vi "HumanDriveButtonBoxReef.vi"(6 "KL":bool, 7 "AB":bool, 8 "IJ":bool, 9 "GH":bool, 10 "EF":bool, 11 "CD":bool) -> (3 "DriveTraj?":bool)   [LabVIEW 2023]
uses:
  HumanBoxReefENUM.ctl
  HumanGlobal.vi
  <vilib>/Rock Robotics/WPI/ThirdParty/JAS_Junk/TrajLib/Trajectory_Library.lvlib
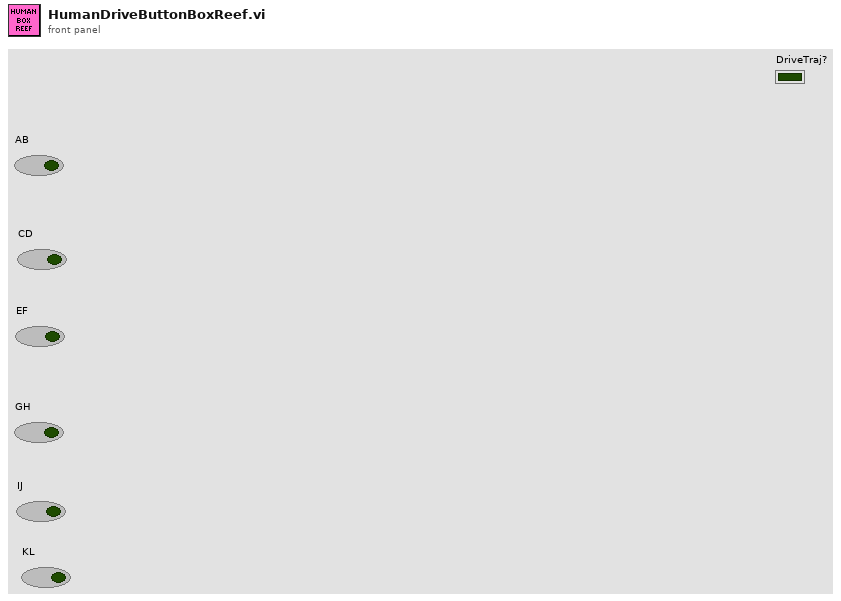
[diagram p1: front panel]
types:
  T1 = typedef "HumanBoxReefENUM.ctl" = enum16{"NoTraj", "A", "B", "C", "D", "E", "F", "G", "H", "I", "J", "K", "L"}
  T2 = typedef "WPI_DriverStationAllianceInfo.ctl" = enum16{"Red", "Blue", "Invalid"}
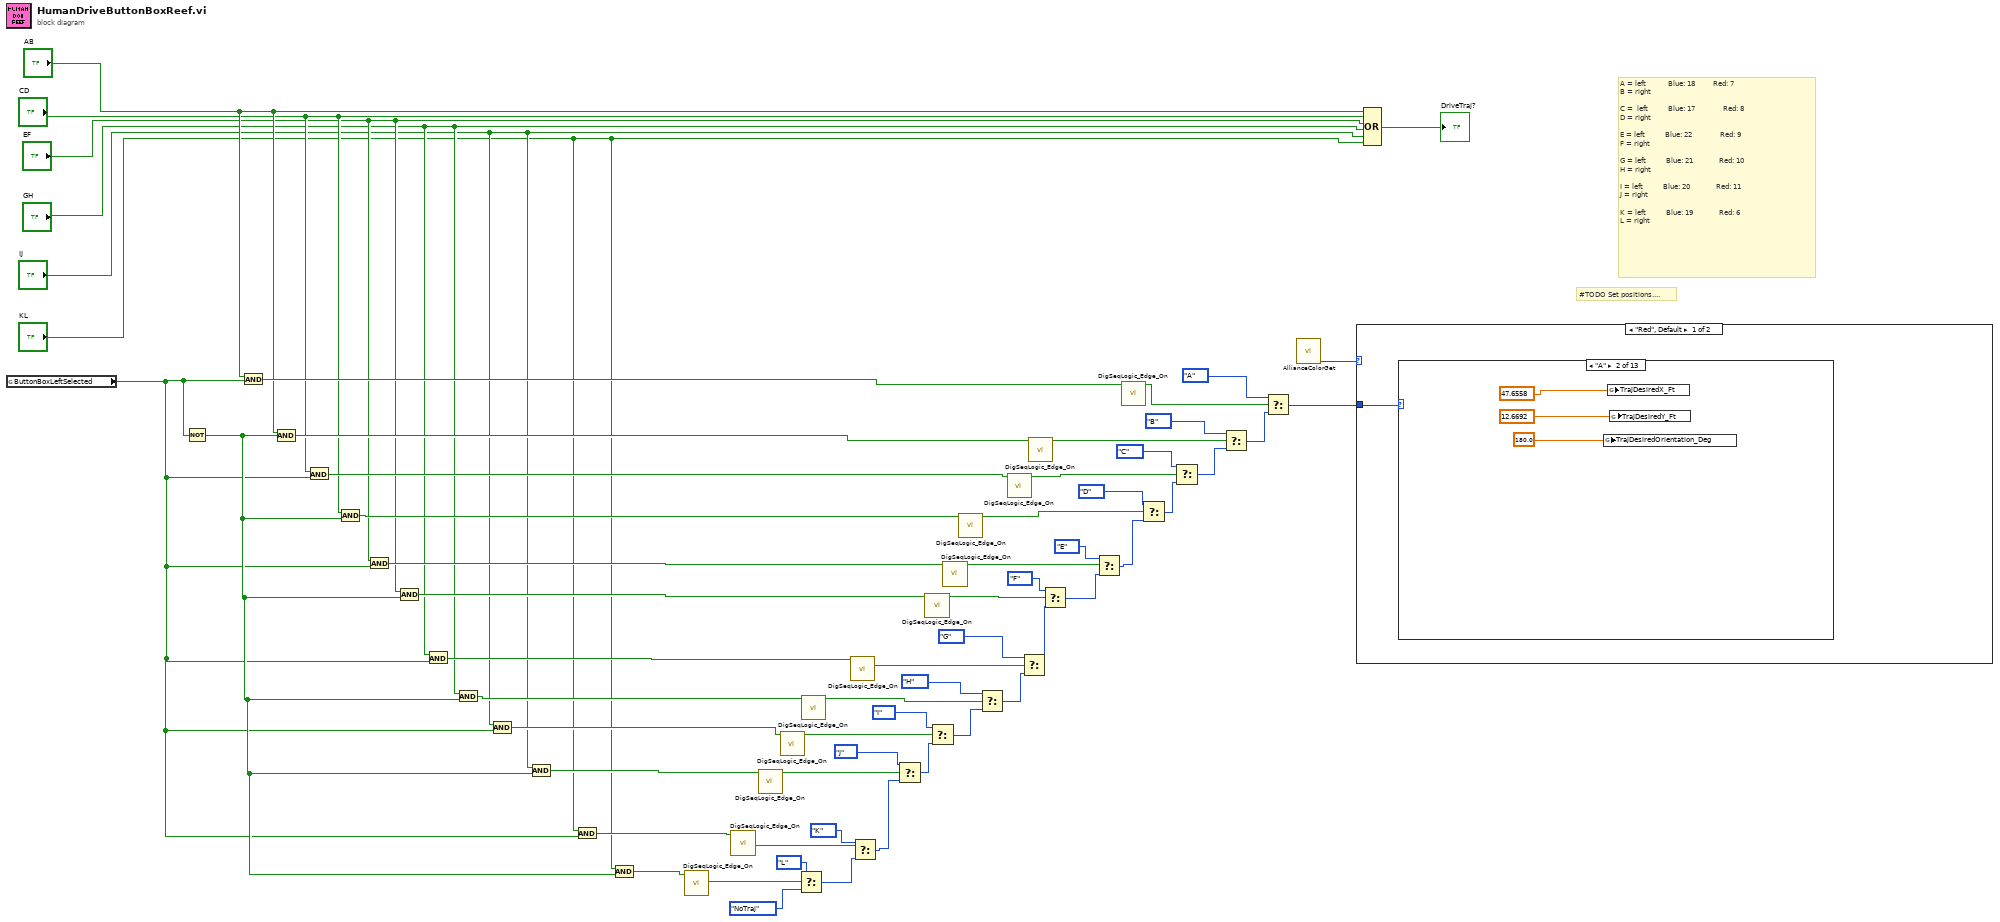
[diagram p0: block diagram]
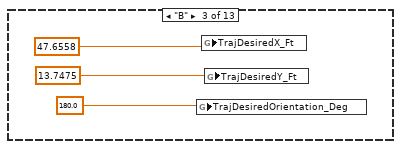
[diagram p3: hidden frame]
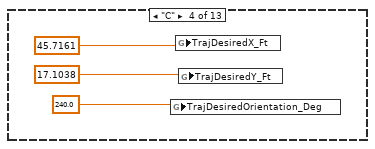
[diagram p4: hidden frame]
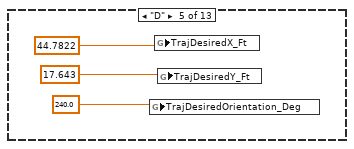
[diagram p5: hidden frame]
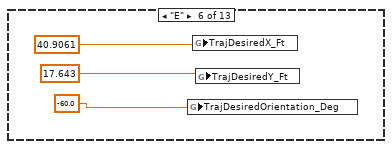
[diagram p6: hidden frame]
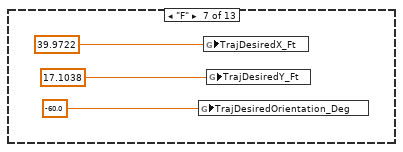
[diagram p7: hidden frame]
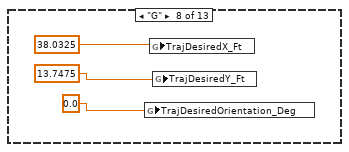
[diagram p8: hidden frame]
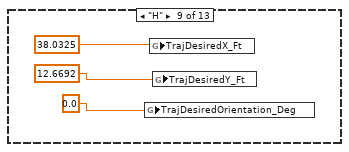
[diagram p9: hidden frame]
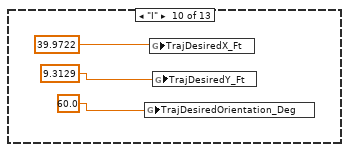
[diagram p10: hidden frame]
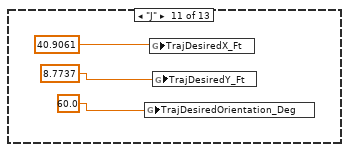
[diagram p11: hidden frame]
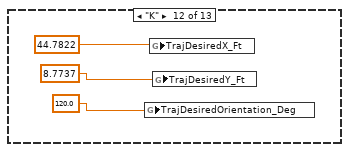
[diagram p12: hidden frame]
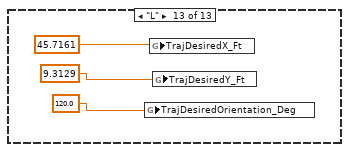
[diagram p13: hidden frame]
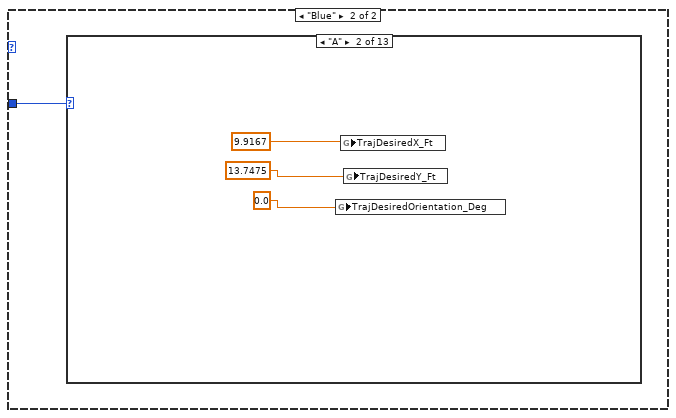
[diagram p14: hidden frame]
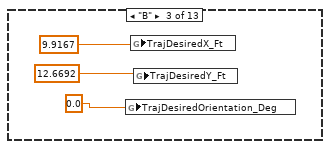
[diagram p16: hidden frame]
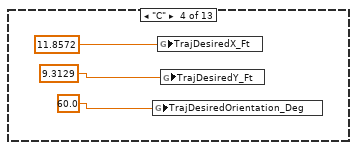
[diagram p17: hidden frame]
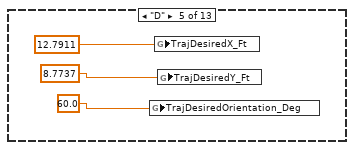
[diagram p18: hidden frame]
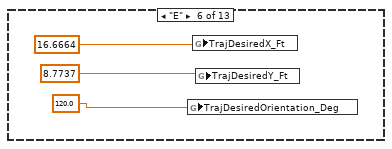
[diagram p19: hidden frame]
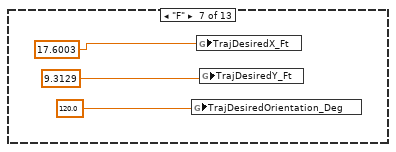
[diagram p20: hidden frame]
diagram:
  # "A = left           Blue: 18         Red: 7\nB = right\n\nC =  left          Blue: 17              Red: 8\nD = right\n\nE = left          Blue: 22              Red: 9\nF = right\n\nG = left          Blue: 21             Red: 10\nH = right\n\nI = left          Blue: 20             Red: 11\nJ = right\n\nK = left          Blue: 19             Red: 6\nL = right"
  # "#TODO Set positions...."
  n1 = global read "HumanGlobal.vi" "ButtonBoxLeftSelected"() -> (w1:bool)
  n2 = Not(x=w1) -> (.not. x?=w2:bool)
  n3 = And(x="AB", y=w1) -> (x .and. y?=w21:bool)
  n4 = And(x="AB", y=w2) -> (x .and. y?=w20:bool)
  n5 = And(x="CD", y=w1) -> (x .and. y?=w19:bool)
  n6 = And(x="CD", y=w2) -> (x .and. y?=w18:bool)
  n7 = And(x="EF", y=w1) -> (x .and. y?=w17:bool)
  n8 = And(x="EF", y=w2) -> (x .and. y?=w16:bool)
  n9 = And(x="GH", y=w1) -> (x .and. y?=w15:bool)
  n10 = And(x="GH", y=w2) -> (x .and. y?=w14:bool)
  n11 = And(x="IJ", y=w1) -> (x .and. y?=w13:bool)
  n12 = And(x="IJ", y=w2) -> (x .and. y?=w12:bool)
  n13 = And(x="KL", y=w1) -> (x .and. y?=w11:bool)
  n14 = And(x="KL", y=w2) -> (x .and. y?=w10:bool)
  n15 = call <vilib>:"DigSeqLogic_Edge_On.vi"("Input"=w10) -> ("On Edge"=w41:bool)  [unwired: 10 in]
  n16 = call <vilib>:"DigSeqLogic_Edge_On.vi"("Input"=w11) -> ("On Edge"=w35:bool)  [unwired: 10 in]
  n17 = call <vilib>:"DigSeqLogic_Edge_On.vi"("Input"=w12) -> ("On Edge"=w34:bool)  [unwired: 10 in]
  n18 = call <vilib>:"DigSeqLogic_Edge_On.vi"("Input"=w13) -> ("On Edge"=w33:bool)  [unwired: 10 in]
  n19 = Select(t=HumanBoxReefENUM."L", s=w41, f=HumanBoxReefENUM."NoTraj" ("t")) -> (s? t:f=w40:T1)
  n20 = call <vilib>:"DigSeqLogic_Edge_On.vi"("Input"=w14) -> ("On Edge"=w32:bool)  [unwired: 10 in]
  n21 = call <vilib>:"DigSeqLogic_Edge_On.vi"("Input"=w15) -> ("On Edge"=w31:bool)  [unwired: 10 in]
  n22 = Select(t=HumanBoxReefENUM."K", s=w35, f=w40) -> (s? t:f=w39:T1)
  n23 = Select(t=HumanBoxReefENUM."J", s=w34, f=w39) -> (s? t:f=w38:T1)
  n24 = call <vilib>:"DigSeqLogic_Edge_On.vi"("Input"=w16) -> ("On Edge"=w59:bool)  [unwired: 10 in]
  n25 = Select(t=HumanBoxReefENUM."I", s=w33, f=w38) -> (s? t:f=w37:T1)
  n26 = call <vilib>:"DigSeqLogic_Edge_On.vi"("Input"=w17) -> ("On Edge"=w53:bool)  [unwired: 10 in]
  n27 = call <vilib>:"DigSeqLogic_Edge_On.vi"("Input"=w18) -> ("On Edge"=w52:bool)  [unwired: 10 in]
  n28 = Select(t=HumanBoxReefENUM."H", s=w32, f=w37) -> (s? t:f=w36:T1)
  n29 = call <vilib>:"DigSeqLogic_Edge_On.vi"("Input"=w19) -> ("On Edge"=w51:bool)  [unwired: 10 in]
  n30 = Select(t=HumanBoxReefENUM."G", s=w31, f=w36) -> (s? t:f=w24:T1)
  n31 = call <vilib>:"DigSeqLogic_Edge_On.vi"("Input"=w20) -> ("On Edge"=w50:bool)  [unwired: 10 in]
  n32 = Select(t=HumanBoxReefENUM."F", s=w59, f=w24) -> (s? t:f=w58:T1)
  n33 = Select(t=HumanBoxReefENUM."E", s=w53, f=w58) -> (s? t:f=w57:T1)
  n34 = call <vilib>:"DigSeqLogic_Edge_On.vi"("Input"=w21) -> ("On Edge"=w22:bool)  [unwired: 10 in]
  n35 = Select(t=HumanBoxReefENUM."D", s=w52, f=w57) -> (s? t:f=w56:T1)
  n36 = Select(t=HumanBoxReefENUM."C", s=w51, f=w56) -> (s? t:f=w55:T1)
  n37 = Select(t=HumanBoxReefENUM."B", s=w50, f=w55) -> (s? t:f=w54:T1)
  n38 = Select(t=HumanBoxReefENUM."A", s=w22, f=w54) -> (s? t:f=w43:T1)
  n39 = call "AllianceColorGet.vi"() -> ("AllianceColor"=w42:T2)  [unwired: 11 in]
  n40 = case shown="\"Red\", Default" w42 {
    tunnel: w43 -> [w60 w97]
    frame "Red", Default {
      n41 = case shown="\"A\"" w60 {
        frame "NoTraj" {
        }
        frame "A" {
          n42 = global write "HumanGlobal.vi" "TrajDesiredOrientation_Deg"(180.0 ("TrajDesiredOrientation_Deg")) -> ()
          n43 = global write "HumanGlobal.vi" "TrajDesiredX_Ft"(47.6558 ("TrajDesiredX_Ft")) -> ()
          n44 = global write "HumanGlobal.vi" "TrajDesiredY_Ft"(12.6692 ("TrajDesiredY_Ft")) -> ()
        }
        frame "B" {
          n45 = global write "HumanGlobal.vi" "TrajDesiredOrientation_Deg"(180.0 ("TrajDesiredOrientation_Deg")) -> ()
          n46 = global write "HumanGlobal.vi" "TrajDesiredX_Ft"(47.6558 ("TrajDesiredX_Ft")) -> ()
          n47 = global write "HumanGlobal.vi" "TrajDesiredY_Ft"(13.7475 ("TrajDesiredY_Ft")) -> ()
        }
        frame "C" {
          n48 = global write "HumanGlobal.vi" "TrajDesiredOrientation_Deg"(240.0 ("TrajDesiredOrientation_Deg")) -> ()
          n49 = global write "HumanGlobal.vi" "TrajDesiredX_Ft"(45.7161 ("TrajDesiredX_Ft")) -> ()
          n50 = global write "HumanGlobal.vi" "TrajDesiredY_Ft"(17.1038 ("TrajDesiredY_Ft")) -> ()
        }
        frame "D" {
          n51 = global write "HumanGlobal.vi" "TrajDesiredOrientation_Deg"(240.0 ("TrajDesiredOrientation_Deg")) -> ()
          n52 = global write "HumanGlobal.vi" "TrajDesiredX_Ft"(44.7822 ("TrajDesiredX_Ft")) -> ()
          n53 = global write "HumanGlobal.vi" "TrajDesiredY_Ft"(17.643 ("TrajDesiredY_Ft")) -> ()
        }
        frame "E" {
          n54 = global write "HumanGlobal.vi" "TrajDesiredOrientation_Deg"(-60.0 ("TrajDesiredOrientation_Deg")) -> ()
          n55 = global write "HumanGlobal.vi" "TrajDesiredX_Ft"(40.9061 ("TrajDesiredX_Ft")) -> ()
          n56 = global write "HumanGlobal.vi" "TrajDesiredY_Ft"(17.643 ("TrajDesiredY_Ft")) -> ()
        }
        frame "F" {
          n57 = global write "HumanGlobal.vi" "TrajDesiredOrientation_Deg"(-60.0 ("TrajDesiredOrientation_Deg")) -> ()
          n58 = global write "HumanGlobal.vi" "TrajDesiredX_Ft"(39.9722 ("TrajDesiredX_Ft")) -> ()
          n59 = global write "HumanGlobal.vi" "TrajDesiredY_Ft"(17.1038 ("TrajDesiredY_Ft")) -> ()
        }
        frame "G" {
          n60 = global write "HumanGlobal.vi" "TrajDesiredOrientation_Deg"(0.0 ("TrajDesiredOrientation_Deg")) -> ()
          n61 = global write "HumanGlobal.vi" "TrajDesiredX_Ft"(38.0325 ("TrajDesiredX_Ft")) -> ()
          n62 = global write "HumanGlobal.vi" "TrajDesiredY_Ft"(13.7475 ("TrajDesiredY_Ft")) -> ()
        }
        frame "H" {
          n63 = global write "HumanGlobal.vi" "TrajDesiredOrientation_Deg"(0.0 ("TrajDesiredOrientation_Deg")) -> ()
          n64 = global write "HumanGlobal.vi" "TrajDesiredX_Ft"(38.0325 ("TrajDesiredX_Ft")) -> ()
          n65 = global write "HumanGlobal.vi" "TrajDesiredY_Ft"(12.6692 ("TrajDesiredY_Ft")) -> ()
        }
        frame "I" {
          n66 = global write "HumanGlobal.vi" "TrajDesiredOrientation_Deg"(60.0 ("TrajDesiredOrientation_Deg")) -> ()
          n67 = global write "HumanGlobal.vi" "TrajDesiredX_Ft"(39.9722 ("TrajDesiredX_Ft")) -> ()
          n68 = global write "HumanGlobal.vi" "TrajDesiredY_Ft"(9.3129 ("TrajDesiredY_Ft")) -> ()
        }
        frame "J" {
          n69 = global write "HumanGlobal.vi" "TrajDesiredOrientation_Deg"(60.0 ("TrajDesiredOrientation_Deg")) -> ()
          n70 = global write "HumanGlobal.vi" "TrajDesiredX_Ft"(40.9061 ("TrajDesiredX_Ft")) -> ()
          n71 = global write "HumanGlobal.vi" "TrajDesiredY_Ft"(8.7737 ("TrajDesiredY_Ft")) -> ()
        }
        frame "K" {
          n72 = global write "HumanGlobal.vi" "TrajDesiredOrientation_Deg"(120.0 ("TrajDesiredOrientation_Deg")) -> ()
          n73 = global write "HumanGlobal.vi" "TrajDesiredX_Ft"(44.7822 ("TrajDesiredX_Ft")) -> ()
          n74 = global write "HumanGlobal.vi" "TrajDesiredY_Ft"(8.7737 ("TrajDesiredY_Ft")) -> ()
        }
        frame "L" {
          n75 = global write "HumanGlobal.vi" "TrajDesiredOrientation_Deg"(120.0 ("TrajDesiredOrientation_Deg")) -> ()
          n76 = global write "HumanGlobal.vi" "TrajDesiredX_Ft"(45.7161 ("TrajDesiredX_Ft")) -> ()
          n77 = global write "HumanGlobal.vi" "TrajDesiredY_Ft"(9.3129 ("TrajDesiredY_Ft")) -> ()
        }
      }
    }
    frame "Blue" {
      n78 = case shown="\"A\"" w97 {
        frame "NoTraj" {
        }
        frame "A" {
          n79 = global write "HumanGlobal.vi" "TrajDesiredOrientation_Deg"(0.0 ("TrajDesiredOrientation_Deg")) -> ()
          n80 = global write "HumanGlobal.vi" "TrajDesiredX_Ft"(9.9167 ("TrajDesiredX_Ft")) -> ()
          n81 = global write "HumanGlobal.vi" "TrajDesiredY_Ft"(13.7475 ("TrajDesiredY_Ft")) -> ()
        }
        frame "B" {
          n82 = global write "HumanGlobal.vi" "TrajDesiredOrientation_Deg"(0.0 ("TrajDesiredOrientation_Deg")) -> ()
          n83 = global write "HumanGlobal.vi" "TrajDesiredX_Ft"(9.9167 ("TrajDesiredX_Ft")) -> ()
          n84 = global write "HumanGlobal.vi" "TrajDesiredY_Ft"(12.6692 ("TrajDesiredY_Ft")) -> ()
        }
        frame "C" {
          n85 = global write "HumanGlobal.vi" "TrajDesiredOrientation_Deg"(60.0 ("TrajDesiredOrientation_Deg")) -> ()
          n86 = global write "HumanGlobal.vi" "TrajDesiredX_Ft"(11.8572 ("TrajDesiredX_Ft")) -> ()
          n87 = global write "HumanGlobal.vi" "TrajDesiredY_Ft"(9.3129 ("TrajDesiredY_Ft")) -> ()
        }
        frame "D" {
          n88 = global write "HumanGlobal.vi" "TrajDesiredOrientation_Deg"(60.0 ("TrajDesiredOrientation_Deg")) -> ()
          n89 = global write "HumanGlobal.vi" "TrajDesiredX_Ft"(12.7911 ("TrajDesiredX_Ft")) -> ()
          n90 = global write "HumanGlobal.vi" "TrajDesiredY_Ft"(8.7737 ("TrajDesiredY_Ft")) -> ()
        }
        frame "E" {
          n91 = global write "HumanGlobal.vi" "TrajDesiredOrientation_Deg"(120.0 ("TrajDesiredOrientation_Deg")) -> ()
          n92 = global write "HumanGlobal.vi" "TrajDesiredX_Ft"(16.6664 ("TrajDesiredX_Ft")) -> ()
          n93 = global write "HumanGlobal.vi" "TrajDesiredY_Ft"(8.7737 ("TrajDesiredY_Ft")) -> ()
        }
        frame "F" {
          n94 = global write "HumanGlobal.vi" "TrajDesiredOrientation_Deg"(120.0 ("TrajDesiredOrientation_Deg")) -> ()
          n95 = global write "HumanGlobal.vi" "TrajDesiredX_Ft"(17.6003 ("TrajDesiredX_Ft")) -> ()
          n96 = global write "HumanGlobal.vi" "TrajDesiredY_Ft"(9.3129 ("TrajDesiredY_Ft")) -> ()
        }
        frame "G" {
          n97 = global write "HumanGlobal.vi" "TrajDesiredOrientation_Deg"(180.0 ("TrajDesiredOrientation_Deg")) -> ()
          n98 = global write "HumanGlobal.vi" "TrajDesiredX_Ft"(19.5408 ("TrajDesiredX_Ft")) -> ()
          n99 = global write "HumanGlobal.vi" "TrajDesiredY_Ft"(12.6692 ("TrajDesiredY_Ft")) -> ()
        }
        frame "H" {
          n100 = global write "HumanGlobal.vi" "TrajDesiredOrientation_Deg"(180.0 ("TrajDesiredOrientation_Deg")) -> ()
          n101 = global write "HumanGlobal.vi" "TrajDesiredX_Ft"(19.5408 ("TrajDesiredX_Ft")) -> ()
          n102 = global write "HumanGlobal.vi" "TrajDesiredY_Ft"(13.7475 ("TrajDesiredY_Ft")) -> ()
        }
        frame "I" {
          n103 = global write "HumanGlobal.vi" "TrajDesiredOrientation_Deg"(240.0 ("TrajDesiredOrientation_Deg")) -> ()
          n104 = global write "HumanGlobal.vi" "TrajDesiredX_Ft"(17.6003 ("TrajDesiredX_Ft")) -> ()
          n105 = global write "HumanGlobal.vi" "TrajDesiredY_Ft"(17.1038 ("TrajDesiredY_Ft")) -> ()
        }
        frame "J" {
          n106 = global write "HumanGlobal.vi" "TrajDesiredOrientation_Deg"(240.0 ("TrajDesiredOrientation_Deg")) -> ()
          n107 = global write "HumanGlobal.vi" "TrajDesiredX_Ft"(16.6664 ("TrajDesiredX_Ft")) -> ()
          n108 = global write "HumanGlobal.vi" "TrajDesiredY_Ft"(17.643 ("TrajDesiredY_Ft")) -> ()
        }
        frame "K" {
          n109 = global write "HumanGlobal.vi" "TrajDesiredOrientation_Deg"(-45.0 ("TrajDesiredOrientation_Deg")) -> ()
          n110 = global write "HumanGlobal.vi" "TrajDesiredX_Ft"(12.2739 ("TrajDesiredX_Ft")) -> ()
          n111 = global write "HumanGlobal.vi" "TrajDesiredY_Ft"(17.4236 ("TrajDesiredY_Ft")) -> ()
        }
        frame "L" {
          n112 = global write "HumanGlobal.vi" "TrajDesiredOrientation_Deg"(-45.0 ("TrajDesiredOrientation_Deg")) -> ()
          n113 = global write "HumanGlobal.vi" "TrajDesiredX_Ft"(11.5114 ("TrajDesiredX_Ft")) -> ()
          n114 = global write "HumanGlobal.vi" "TrajDesiredY_Ft"(16.6611 ("TrajDesiredY_Ft")) -> ()
        }
      }
    }
  }
  n115 = Compound Arithmetic op=OR("AB", "CD", "EF", "GH", "IJ", "KL") -> (→"DriveTraj?":bool)
